vi "Lab 5-2 Labview code.vi"() -> ()   [LabVIEW 2021]
uses:
  <vilib>/Analysis/NI_AALBase.lvlib
  <vilib>/Analysis/NI_AALPro.lvlib
panel:
  out "PTT Std":dbl
  out "PTT Mean":dbl
  out "RRV Std":dbl
  out "RRV Mean":dbl
  out "PTT Graph":cluster{"Y":dbl[], "Y":dbl[]}[](graph)
  out "RRV Graph":cluster{"Y":dbl[], "Y":dbl[]}[](graph)
  out "Filtered PPG Graph":dynamicdata(graph)
  out "Filtered ECG Graph":dynamicdata(graph)
  out "Raw PPG Graph":dynamicdata(graph)
  out "Raw ECG Graph":dynamicdata(graph)
  in  "stop (F)":bool
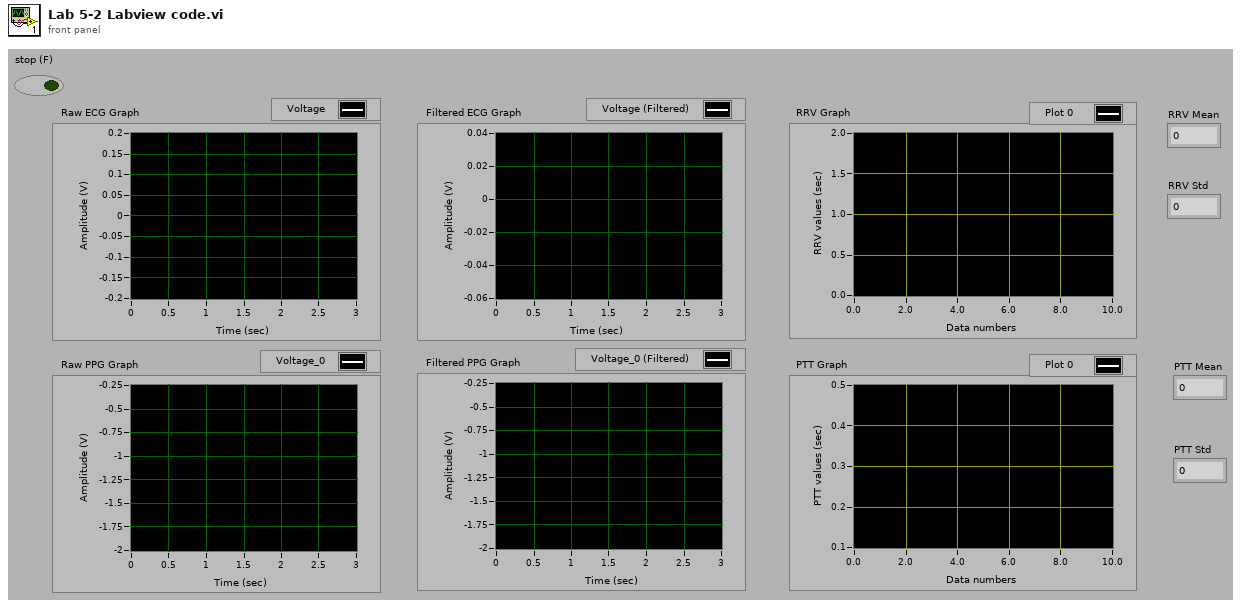
[diagram p1: front panel]
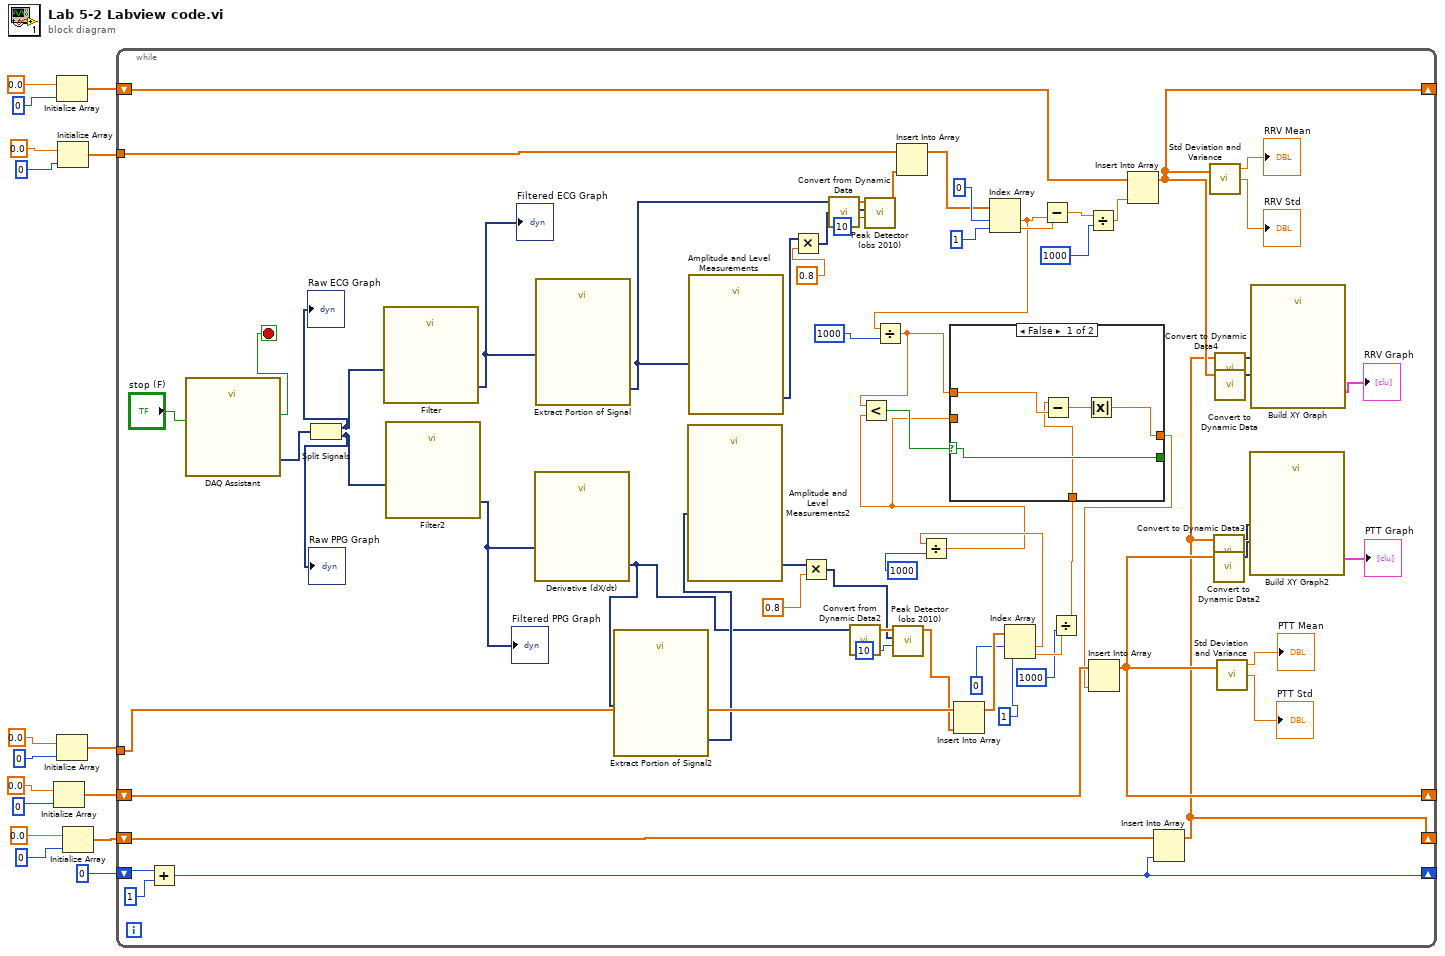
[diagram p0: block diagram]
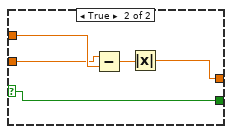
[diagram p2: hidden frame]
diagram:
  n1 = Initialize Array(0.0, 0) -> (w7:dbl[])
  n2 = Initialize Array(0.0, 0) -> (w8:dbl[])
  n3 = Initialize Array(0.0, 0) -> (w4:dbl[])
  n4 = Initialize Array(0.0, 0) -> (w5:dbl[])
  n5 = Initialize Array(0.0 ("element"), 0 ("dimension size")) -> (w1:dbl[])
  n6 = while {
    shift-right: [w65] -> _
    shift-left: w8 -> [w72]
    shift-right: [w63] -> _
    shift-left: w7 -> [w71]
    tunnel: w5 -> [w68]
    tunnel: w4 -> [w67]
    shift-right: [w60] -> _
    shift-left: 0 -> [w70]
    shift-right: [w58] -> _
    shift-left: w1 -> [w61]
    stop <- w47 stop-if-true
    n7 = Add(x=w70, y=1) -> (x+y=w60:i32)
    n8 = call "DAQ Assistant"("stop (F)"="stop (F)") -> ("data"=w46:dynamicdata, "stopped"=w47:bool)  [unwired: 15 in, 2 out]
    n9 = Split Signals(w46) -> (w80:dynamicdata, w79:dynamicdata)  [unwired: 2 in]
    "Raw ECG Graph" <- w80
    "Raw PPG Graph" <- w79
    n10 = call "Filter"("Signal"=w80) -> ("Filtered Signal"=w55:dynamicdata)  [unwired: 9 in, 1 out]
    "Filtered ECG Graph" <- w55
    n11 = call "Filter2"("Signal"=w79) -> ("Filtered Signal"=w54:dynamicdata)  [unwired: 9 in, 1 out]
    "Filtered PPG Graph" <- w54
    n12 = call "Derivative (dX/dt)"("Signals"=w54) -> ("Result"=w17:dynamicdata)  [unwired: 5 in, 1 out]
    n13 = call "Extract Portion of Signal"("Signals"=w55) -> ("Section"=w52:dynamicdata)  [unwired: 9 in, 1 out]
    n14 = call "Extract Portion of Signal2"("Signals"=w17) -> ("Section"=w53:dynamicdata)  [unwired: 9 in, 1 out]
    n15 = call "Amplitude and Level Measurements2"("Signals"=w53) -> ("Positive Peak"=w20:dynamicdata)  [unwired: 12 in, 2 out]
    n16 = call "Amplitude and Level Measurements"("Signals"=w52) -> ("Positive Peak"=w44:dynamicdata)  [unwired: 13 in, 1 out]
    n17 = Multiply(x=w44, y=0.8) -> (x*y=w42:dynamicdata)
    n18 = Multiply(x=w20, y=0.8) -> (x*y=w18:dynamicdata)
    n19 = call "Convert from Dynamic Data"("Dynamic Data Type"=w52) -> ("Array"=w51:dbl[])  [unwired: 3 in]
    n20 = call "Convert from Dynamic Data2"("Dynamic Data Type"=w17) -> ("Array"=w50:dbl[])  [unwired: 3 in]
    n21 = call <vilib>:"Peak Detector (obs 2010).vi"("width"=10, "threshold"=w42, "X"=w51) -> ("Locations"=w37:dbl[])  [unwired: 4 in, 4 out]
    n22 = call <vilib>:"Peak Detector (obs 2010).vi"("width"=10, "threshold"=w18, "X"=w50) -> ("Locations"=w66:dbl[])  [unwired: 4 in, 4 out]
    n23 = Insert Into Array(array=w68, new element=w37) -> (w27:dbl[])  [unwired: 1 in]
    n24 = Insert Into Array(array=w67, new element=w66) -> (w30:dbl[])  [unwired: 1 in]
    n25 = Index Array(array=w27, index #1=0 ("width"), index #2=1 ("width")) -> (element #1=w31:dbl, element #2=w32:dbl)
    n26 = Divide(x=w31, y=1000) -> (x/y=w25:dbl)
    n27 = Index Array(array=w30, index #1=0 ("width"), index #2=1 ("width")) -> (element #1=w28:dbl, element #2=w24:dbl)
    n28 = Divide(x=w28, y=1000) -> (x/y=w21:dbl)
    n29 = Less?(x=w25, y=w21) -> (x < y?=w35:bool)
    n30 = Subtract(x=w32, y=w31) -> (x-y=w41:dbl)
    n31 = Divide(x=w24, y=1000) -> (x/y=w22:dbl)
    n32 = case shown="False" w35 {
      selector: w35 -> [w85 w90]
      tunnel: [w81 w86] -> w49
      tunnel: [w85 w90] -> _
      tunnel: w25 -> [w84 w89]
      tunnel: w22 -> [w83 _]
      tunnel: w21 -> [_ w88]
      frame False {
        n33 = Subtract(x=w83, y=w84) -> (x-y=w82:dbl)
        n34 = Absolute Value(x=w82) -> (abs(x)=w81:dbl)
      }
      frame True {
        n35 = Subtract(x=w88, y=w89) -> (x-y=w87:dbl)
        n36 = Absolute Value(x=w87) -> (abs(x)=w86:dbl)
      }
    }
    n37 = Divide(x=w41, y=1000) -> (x/y=w38:dbl)
    n38 = Insert Into Array(array=w71, new element=w49) -> (w63:dbl[])  [unwired: 1 in]
    n39 = Insert Into Array(array=w72, new element=w38) -> (w65:dbl[])  [unwired: 1 in]
    n40 = Insert Into Array(array=w61, new element=w60) -> (w58:dbl[])  [unwired: 1 in]
    n41 = call <vilib>:"Std Deviation and Variance.vi"("X"=w65) -> ("mean"=→"RRV Mean":dbl, "standard deviation"=→"RRV Std":dbl)  [unwired: 1 in, 1 out]
    n42 = call "Convert to Dynamic Data3"("Array"=w58) -> ("Dynamic Data Type"=w59:dynamicdata)  [unwired: 3 in]
    n43 = call "Convert to Dynamic Data2"("Array"=w63) -> ("Dynamic Data Type"=w62:dynamicdata)  [unwired: 3 in]
    n44 = call "Convert to Dynamic Data4"("Array"=w58) -> ("Dynamic Data Type"=w57:dynamicdata)  [unwired: 3 in]
    n45 = call "Convert to Dynamic Data"("Array"=w65) -> ("Dynamic Data Type"=w64:dynamicdata)  [unwired: 3 in]
    n46 = call <vilib>:"Std Deviation and Variance.vi"("X"=w63) -> ("mean"=→"PTT Mean":dbl, "standard deviation"=→"PTT Std":dbl)  [unwired: 1 in, 1 out]
    n47 = call "Build XY Graph2"("Y Input"=w62, "X Input"=w59) -> ("XY Graph"=→"PTT Graph":cluster{"Y":dbl[], "Y":dbl[]}[])  [unwired: 8 in, 1 out]
    n48 = call "Build XY Graph"("Y Input"=w64, "X Input"=w57) -> ("XY Graph"=→"RRV Graph":cluster{"Y":dbl[], "Y":dbl[]}[])  [unwired: 8 in, 1 out]
  }
